vi "pp2_arraySelect_test.vi"() -> ()   [LabVIEW 2013]
panel:
  out "Column Labels":string[][](table)
  out "Table Control":string[][](table)
  out "Session List":u8[][](array[numeric])
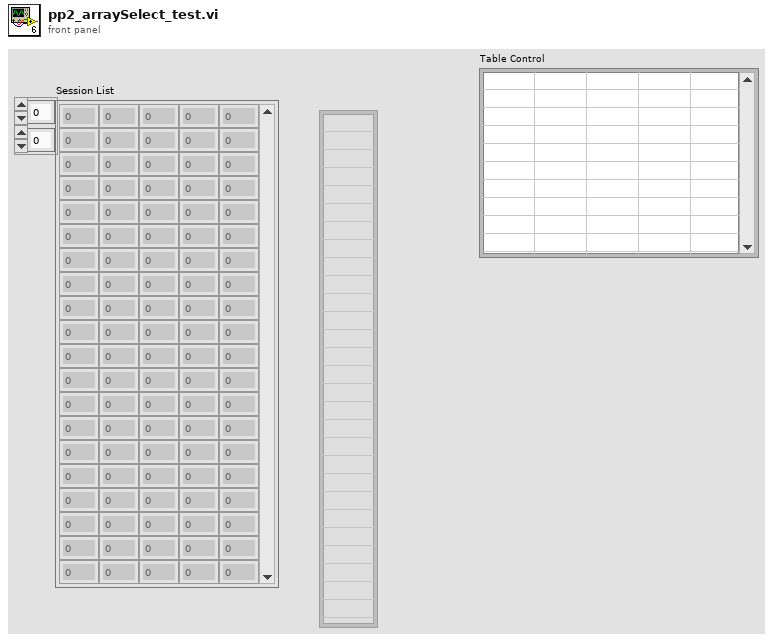
[diagram p1: front panel]
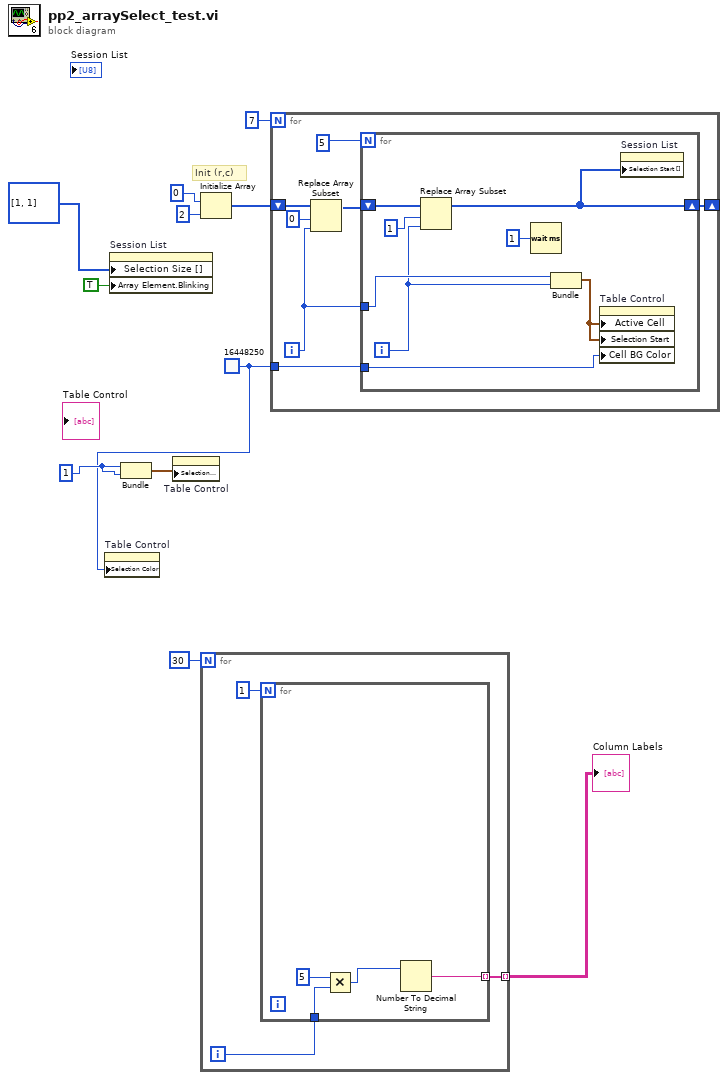
[diagram p0: block diagram]
diagram:
  w5 = 1 ("index")
  w4 = u32 16448250
  # "Init (r,c)"
  n1 = property on="Table Control" class="Tbl (strict)"("Selection Color"=w4) -> ()  [unwired: 2 in, 2 out]
  n2 = property on="Session List" class="Arr (strict)"("Selection Size []"=u32[] [1, 1] ("Selection Size[]"), "Array Element.Blinking"=TRUE) -> ()  [unwired: 2 in, 2 out]
  n3 = Bundle("index"=w5, "index"=w5) -> (w6:cluster{"index":i32, "index":i32})  [unwired: 1 in]
  n4 = property on="Table Control" class="Tbl (strict)"("Selection Size"=w6) -> ()  [unwired: 2 in, 2 out]
  n5 = Initialize Array(0, 2 ("dimension size")) -> (w9:i32[])
  n6 = for {
    N: 30 -> [_]
    tunnel: [w14] -> w2 mode=indexing
    i -> [w12]
    n7 = for {
      N: 1 -> [_]
      tunnel: [w16] -> w14 mode=indexing
      tunnel: w12 -> [w15]
      n8 = Multiply(x=5, y=w15) -> (x*y=w17:i32)
      n9 = Number To Decimal String(number=w17) -> (decimal integer string=w16:string)  [unwired: 1 in]
    }
  }
  "Column Labels" <- w2
  n10 = for {
    N: 7 -> [_]
    shift-right: [w21] -> _
    shift-left: w9 -> [w24]
    tunnel: w4 -> [w19]
    i -> [w20]
    n11 = Replace Array Subset(array=w24, new element=w20, index=0) -> (w23:i32[])
    n12 = for {
      N: 5 -> [_]
      shift-right: [w30] -> w21
      shift-left: w23 -> [w32]
      tunnel: w20 -> [w29]
      tunnel: w19 -> [w27]
      i -> [w28]
      n13 = Replace Array Subset(array=w32, new element=w28, index=1) -> (w30:i32[])
      n14 = Wait (ms)(milliseconds to wait=u32 1) -> ()  [unwired: 1 out]
      n15 = Bundle(w29, w28) -> (w26:cluster{i32, i32})  [unwired: 1 in]
      n16 = property on="Table Control" class="Tbl (strict)"("Active Cell"=w26, "Selection Start"=w26, "Cell BG Color"=w27) -> ()  [unwired: 2 in, 2 out]
      n17 = property on="Session List" class="Arr (strict)"("Selection Start []"=w30) -> ()  [unwired: 2 in, 2 out]
    }
  }
